vi "GUIAS CURVAS EM FUNÇÃO DO RAIO-6.vi"() -> ()   [LabVIEW 2014]
uses:
  <vilib>/Platform/TimedLoop/XDataNode/timing_clust.ctl
  <vilib>/Platform/TimedLoop/XDataNode/nitl_modes.ctl
  <vilib>/Platform/TimedLoop/XDataNode/wakeup.ctl
  <vilib>/Instr/_visa.llb/VISA Configure Serial Port (Instr).vi
  <vilib>/Platform/TimedLoop/XDataNode/XDataNode.xnode
  <userlib>/Newport ESP301/Newport ESP301.lvlib
  <vilib>/Platform/TimedLoop/XDataNode/XDNodeRunTimeDep.lvlib
panel:
  in  "Aceleracao":dbl=2.0
  in  "Velocity":dbl=3.0
  out "Yin":dbl format="%.6g"
  out "Xin":dbl format="%.6g"
  out "Raio":dbl
  out "PROGRESSÃO":i32
  in  "Raios":dbl[](array[numeric])=[40.0, 60.0, 80.0, 100.0, 120.0, 140.0, 180.0]
  in  "N_Guias":dbl=7.0
  in  "Iniciar":bool
  in  "L":dbl=10.0 format="%.1f"
  in  "In.Curva":dbl=2.0
  out "d (um)":dbl
  in  "Distância (um)":dbl=50.0
  in  "Stop Button":bool
  out "X (mm)":dbl format="%.2g"
  out "Y (um)":dbl format="%.1f"
  out "XY Graph":cluster{dbl[], dbl[]}(graph)={[0.0, 0.0, 0.0, 0.0, 0.0, 0.0, 0.0, 0.0, 0.0, 0.0, 0.0, 0.0, 0.0, 0.0, 0.0, 0.0, 0.0, 0.0, 0.0, 0.0, 0.0, 0.0, 0.0, 0.0, 0.0, 0.0, 0.0, 0.0, 0.0, 0.0, 0.0, 0.0, 0.0, 0.0, 0.0, 0.0, 0.0, 0.0, 0.0, 0.0, 0.0, 0.0, 0.0, 0.0, 0.0, 0.0, 0.0, 0.0, 0.0, 0.0, 0.0, 0.0, 0.0, 0.0, 0.0, 0.0, 0.0, 0.0, 0.0, 0.0, 0.0, 0.0, 0.0, 0.0, 0.0, 0.0, 0.0, 0.0, 0.0, 0.0, 0.0, 0.0, 0.0, 0.0, 0.0, 0.0], [4600.0, 4600.0, 4600.0, 4600.0, 4600.0, 4600.0, 4600.0, 4600.0, 4600.0, 4600.0, 4600.0, 4600.0, 4600.0, 4600.0, 4600.0, 4600.0, 4600.0, 4600.0, 4600.0, 4600.0, 4600.0, 4600.0, 4600.0, 4600.0, 4600.0, 4600.0, 4600.0, 4690.0, 4802.5, 4800.5, 4799.5, 4799.5, 4799.5, 4800.0, 4800.0, 4800.0, 4800.0, 4800.0, 4800.0, 4800.0, 4800.0, 4800.0, 4800.0, 4800.0, 4995.5, 5001.5, 5000.5, 5000.0, 5000.0, 4999.5, 4999.5, 5000.0, 5000.0, 5000.0, 5000.0, 5000.0, 5000.0, 5000.0, 5000.0, 5000.0, 5000.0, 5000.0, 5000.0, 5000.0, 5000.0, 5000.0, 5000.0, 5000.0, 5000.0, 5000.0, 5000.0, 5000.0, 5000.0, 5000.0, 5000.0, 5000.0]}
  in  "Refresh Button":bool
  # "Inicio curva"
  # "Tam.amostra (mm)"
  # "Núm.guias"
  # "Raio (mm)"
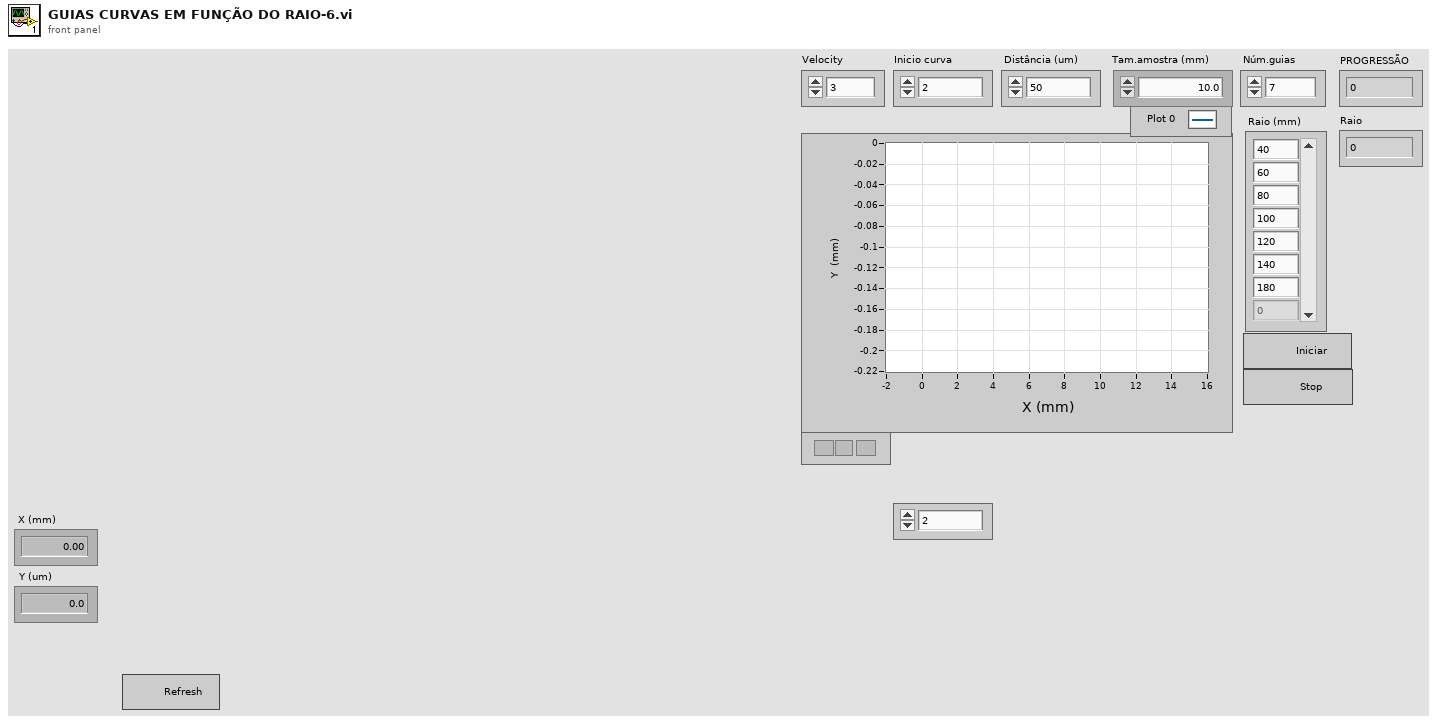
[diagram p1: front panel]
types:
  T1 = typedef "XDNodeRunTimeDep.lvlib/timing_clust.ctl" = cluster{"Expected End [f-1]":u64, "Actual End [f-1]":u64, "Finished Late? [f-1]":bool, "Expected End [i-1]":u64, "Actual End [i-1]":u64, "Finished Late? [i-1]":bool, "Expected Start [i]":u64, "Actual Start [i]":u64, "Expected Start [f]":u64, "Actual Start [f]":u64, "Source Name":string, "Structure Name":string, "Period":i64, "Deadline":i64, "Offset":i64, "Start":i64, "Priority":i32, "Timeout":i32, "Mode":T2, "Wakeup Reason":T3, "Error":errorcluster, "Source Type":string, "Secondary Source Type":string, "Global End Time":u64, "Global Start Time":u64, "Frame Duration":u64, "Iteration Duration":u64, "Assigned CPU":i32, "I/O Scan Engine Mode":u32}
  T2 = typedef "XDNodeRunTimeDep.lvlib/nitl_modes.ctl" = enum32{"No Change", "Process missed periods, maintain original phase", "Discard missed periods, maintain original phase", "Process missed periods, ignore original phase", "Discard missed periods, ignore original phase"}
  T3 = typedef "XDNodeRunTimeDep.lvlib/wakeup.ctl" = enum32{"Normal", "Aborted", "Asynchronous wakeup", "Timing source error", "Timed loop error", "Timeout"}
  T4 = cluster{"Axis1 moving":bool, "Axis2 moving":bool, "Axis3 moving":bool, "Axis4 moving":bool, "Motor Power of at least one axis":bool, "Reserved":bool, "Reserved":bool, "Reserved":bool, "Axis5 moving 2":bool, "Axis6 moving 2":bool, "Reserved":bool, "Reserved":bool, "Motor Power of at least one axis":bool, "Reserved":bool, "Reserved":bool, "Reserved":bool}
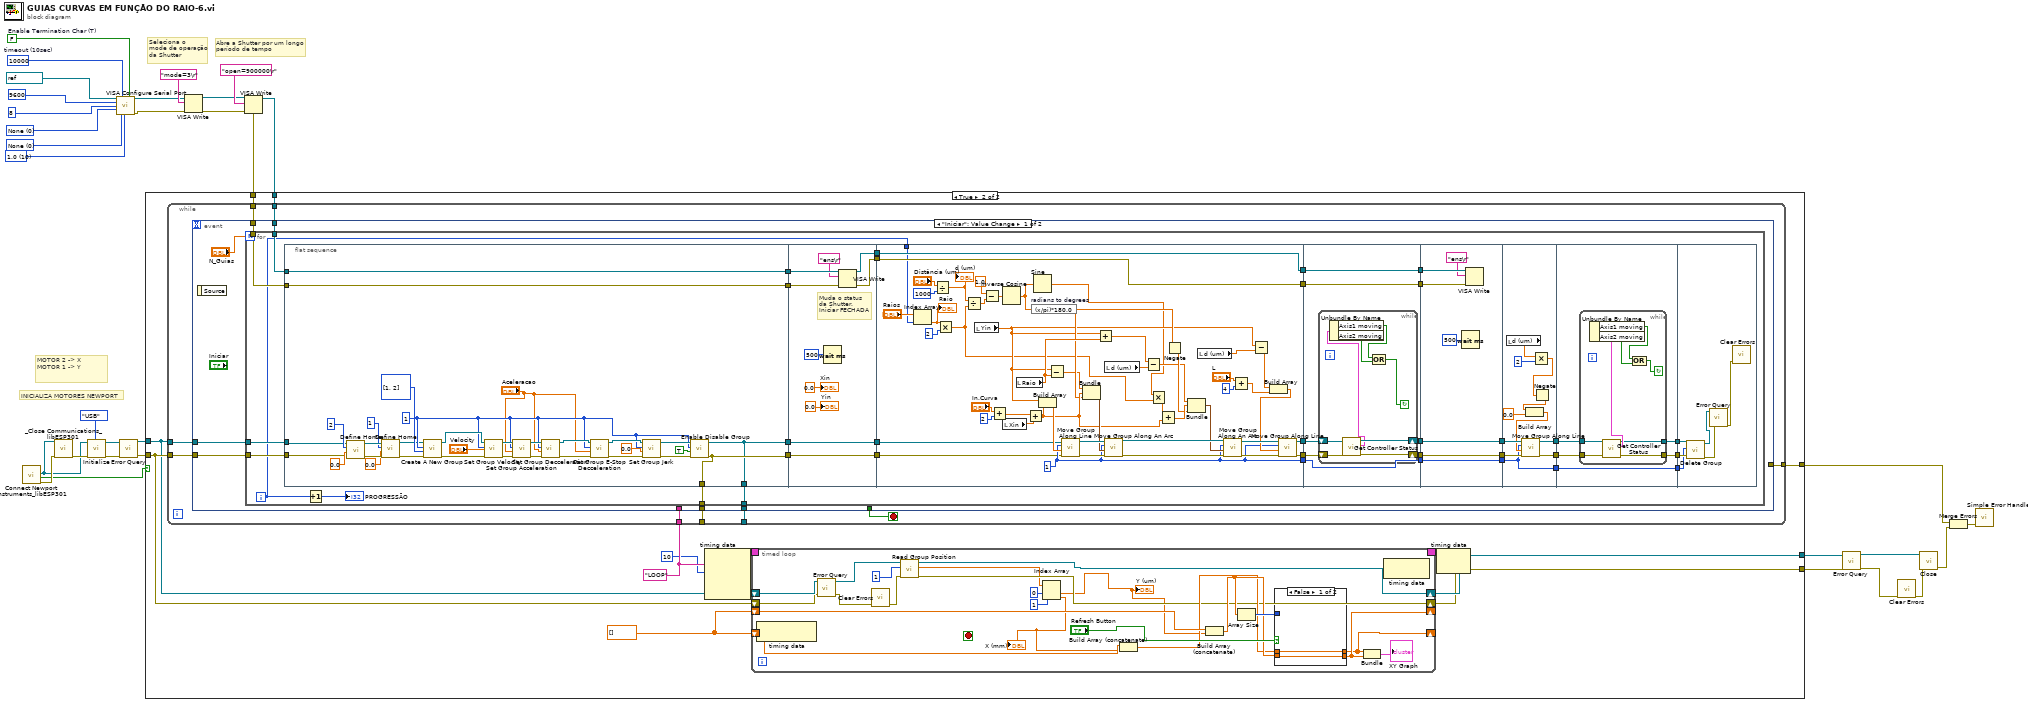
[diagram p0: block diagram]
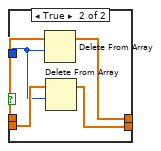
[diagram p3: hidden frame]
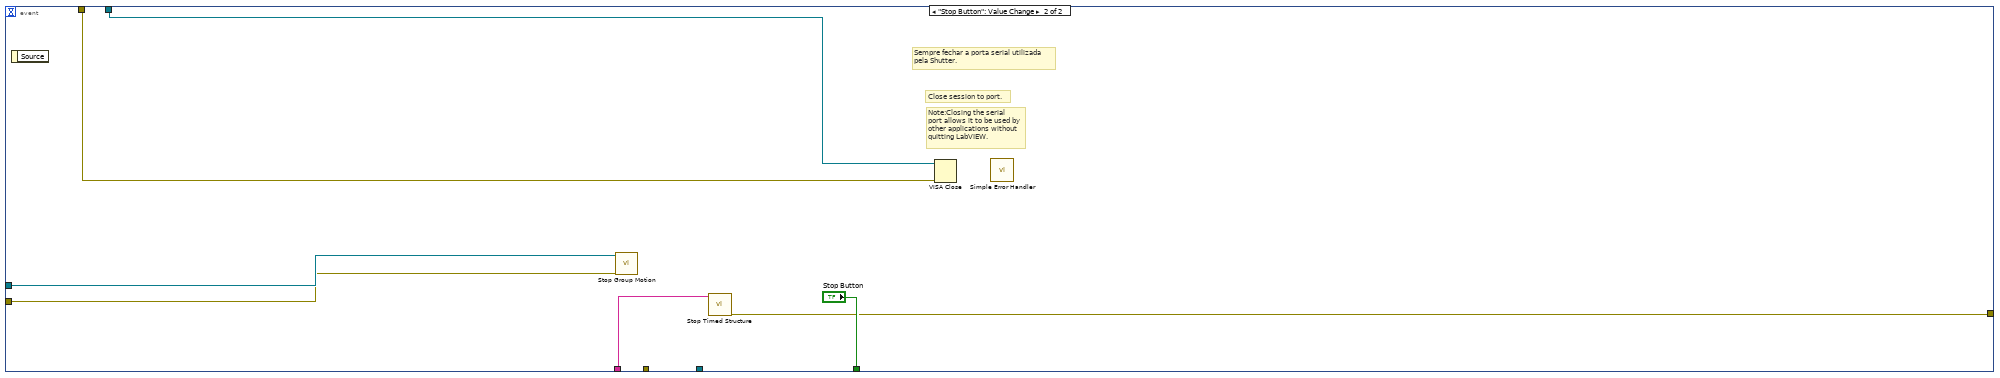
[diagram p4: hidden frame]
diagram:
  w9 = u16 0 items=["None", "Odd", "Even", "Mark", "Space"] ("parity")
  w12 = u16 10 items=["1.0"=10, "1.5"=15, "2.0"=20] ("stop bits")
  w13 = u16 0 items=["None"=0, "XON/XOFF"=1, "RTS/CTS"=2, "DTR/DSR"=4] ("flow control")
  w11 = FALSE  # Enable Termination Char (T)
  w10 = u32 10000  # timeout (10sec)
  # "Abre a Shutter por um longo\nperíodo de tempo"
  # "Seleciona o \nmode de operação\nda Shutter"
  # "MOTOR 2 -> X\nMOTOR 1 -> Y"
  # "INICIALIZA MOTORES NEWPORT"
  n1 = call <userlib>:"Connect Newport Instruments_libESP301.vi"() -> ("error (duplicate)"=w31:errorcluster, "Connected"=w20:bool, "VISA resource name (duplicate)"=w30:refnum<visa-resource-name>)  [unwired: 7 in, 2 out]
  n2 = call <userlib>:"_Close Communications_libESP301.vi"("Instrument Channel"=w30, "error in (no error)"=w31) -> ("error out"=w33:errorcluster)  [unwired: 13 in]
  n3 = call <userlib>:"Initialize.vi"("VISA resource name"=w30, "error in (no error)"=w33, "Serial Link (RS232)"=enum16{"RS232", "USB"}."USB") -> ("VISA resource name out"=w29:refnum<visa-resource-name>, "error out"=w28:errorcluster)  [unwired: 6 in]
  n4 = call-poly "VISA Configure Serial Port"("VISA resource name"=refnum<visa-resource-name> "COM6", "timeout (10sec)"=w10, "Enable Termination\nChar (T)"=w11, "baud rate (9600)"=u32 9600 ("baud rate"), "data bits (8)"=u16 8 ("data bits"), "parity (0:none)"=w9, "stop bits (10: 1 bit)"=w12, "flow control (0:none)"=w13) -> ("VISA resource name out"=w5:refnum<visa-resource-name>, "error out"=w4:errorcluster)  [unwired: 6 in]
  n5 = call <userlib>:"Error Query.vi"("error in (no error)"=w28, "VISA resource name"=w29) -> ("error out"=w17:errorcluster, "VISA resource name out"=w18:refnum<visa-resource-name>)  [unwired: 2 in, 2 out]
  n6 = VISA Write(VISA resource name=w5, write buffer="mode=3\r", error in (no error)=w4) -> (VISA resource name out=w2:refnum<visa-resource-name>, error out=w1:errorcluster)  [unwired: 1 out]
  n7 = VISA Write(VISA resource name=w2, write buffer="open=900000\r", error in (no error)=w1) -> (VISA resource name out=w21:refnum<visa-resource-name>, error out=w19:errorcluster)  [unwired: 1 out]
  n8 = case shown="True" w20 {
    tunnel: [w35 w47] -> w16
    tunnel: [w34 w46] -> w15
    tunnel: w18 -> [w35 w36]
    tunnel: w17 -> [w34 w37]
    tunnel: [_ w44] -> w24
    tunnel: w21 -> [_ w43]
    tunnel: w19 -> [_ w42]
    frame False {
    }
    frame True {
      w38 = dbl[] []
      w45 = "LOOP" ("Structure Name")
      n9 = while {
        tunnel: w37 -> [w92]
        tunnel: w36 -> [w91]
        tunnel: w45 -> [w89]
        tunnel: [w88] -> w44
        tunnel: w43 -> [w87]
        tunnel: w42 -> [w86]
        tunnel: [w85] -> _
        tunnel: [w84] -> _
        stop <- w90 stop-if-true
        n10 = event shown="[0] \"Iniciar\": Value Change" {
          selector: _ -> [_ _]
          dyn-events: _ -> [_ _]
          timeout: _ -> [_ _]
          tunnel: w92 -> [w99 w280]
          tunnel: w91 -> [w98 w281]
          tunnel: [_ "Stop Button"] -> w90
          tunnel: w89 -> [_ w284]
          tunnel: [_ w283] -> w88
          tunnel: w87 -> [w96 w282]
          tunnel: w86 -> [w95 w279]
          tunnel: [w94 _] -> w85
          tunnel: [w93 _] -> w84
          event "Iniciar": Value Change {
            n11 = event-data() -> ()  [unwired: 1 in, 1 out]
            n12 = for {
              N: "N_Guias" -> [_]
              tunnel: w99 -> [w132]
              tunnel: w98 -> [w131]
              tunnel: w96 -> [w129]
              tunnel: w95 -> [w111]
              tunnel: [w101] -> w94
              tunnel: [w100] -> w93
              i -> [w110]
              n13 = flat-sequence {
                tunnel: w111 -> [w165]
                tunnel: w129 -> [w166]
                tunnel: w131 -> [w139]
                tunnel: w132 -> [w138]
                tunnel: [w137] -> w109
                tunnel: [w136] -> w108
                tunnel: [w166] -> w107
                tunnel: [w165] -> w106
                tunnel: [w137] -> w101
                tunnel: [w136] -> w100
                tunnel: [w170] -> w134
                tunnel: [w171] -> w133
                tunnel: [w174] -> w119
                tunnel: [w173] -> w116
                tunnel: w109 -> [w170]
                tunnel: w108 -> [w171]
                tunnel: w107 -> [w175]
                tunnel: w106 -> [w172]
                tunnel: w134 -> [w179]
                tunnel: w133 -> [w180]
                tunnel: w110 -> [w188]
                tunnel: [w193] -> w126
                tunnel: [w192] -> w125
                tunnel: [w191] -> w122
                tunnel: w119 -> [w189]
                tunnel: [w190] -> w117
                tunnel: w116 -> [w190]
                tunnel: [w189] -> w115
                tunnel: [w233] -> w127
                tunnel: w126 -> [w233]
                tunnel: w125 -> [w229]
                tunnel: [w227] -> w124
                tunnel: w122 -> [w230]
                tunnel: [w228] -> w121
                tunnel: [w232] -> w118
                tunnel: w117 -> [w232]
                tunnel: w115 -> [w231]
                tunnel: [w231] -> w114
                tunnel: [w248] -> w128
                tunnel: w127 -> [w248]
                tunnel: w124 -> [w247]
                tunnel: [w247] -> w123
                tunnel: w121 -> [w246]
                tunnel: [w246] -> w120
                tunnel: w118 -> [w245]
                tunnel: w114 -> [w244]
                tunnel: w128 -> [w249]
                tunnel: w123 -> [w259]
                tunnel: w120 -> [w258]
                tunnel: [w252] -> w113
                tunnel: [w251] -> w112
                tunnel: [w249] -> w102
                tunnel: w113 -> [w264]
                tunnel: w112 -> [w263]
                tunnel: [w262] -> w105
                tunnel: [w261] -> w104
                tunnel: [w260] -> w103
                tunnel: w102 -> [w260]
                tunnel: w105 -> [w278]
                tunnel: w104 -> [w277]
                tunnel: w103 -> [w276]
                frame #0 {
                  w148 = 1 ("Group #")
                  n14 = call <userlib>:"Define Home.vi"("error in (no error)"=w138, "Home Position (0 units)"=0.0, "Axis (1)"=2 ("y"), "VISA resource name"=w139) -> ("error out"=w146:errorcluster, "VISA resource name out"=w147:refnum<visa-resource-name>)  [unwired: 2 in]
                  n15 = call <userlib>:"Define Home.vi"("error in (no error)"=w146, "Home Position (0 units)"=0.0, "Axis (1)"=1, "VISA resource name"=w147) -> ("error out"=w140:errorcluster, "VISA resource name out"=w141:refnum<visa-resource-name>)  [unwired: 2 in]
                  n16 = call <userlib>:"Create A New Group.vi"("error in (no error)"=w140, "Axis Number"=i32[] [1, 2], "Group Number (1)"=w148, "VISA resource name"=w141) -> ("error out"=w162:errorcluster, "VISA resource name out"=w163:refnum<visa-resource-name>)  [unwired: 2 in]
                  n17 = call <userlib>:"Set Group Velocity.vi"("error in (no error)"=w162, "Velocity (units/s)"="Velocity", "Group Number (1)"=w148, "VISA resource name"=w163) -> ("error out"=w157:errorcluster, "VISA resource name out"=w160:refnum<visa-resource-name>)  [unwired: 2 in]
                  n18 = call <userlib>:"Set Group Acceleration.vi"("error in (no error)"=w157, "Acceleration (0 units/s²)"="Aceleracao", "Group Number (1)"=w148, "VISA resource name"=w160) -> ("error out"=w158:errorcluster, "VISA resource name out"=w159:refnum<visa-resource-name>)  [unwired: 2 in]
                  n19 = call <userlib>:"Set Group Decceleration.vi"("error in (no error)"=w158, "Decceleration (0 units/s²)"="Aceleracao", "Group Number (1)"=w148, "VISA resource name"=w159) -> ("error out"=w153:errorcluster, "VISA resource name out"=w156:refnum<visa-resource-name>)  [unwired: 2 in]
                  n20 = call <userlib>:"Set Group E-Stop Decceleration.vi"("error in (no error)"=w153, "E-Stop Decceleration (0 units/s²)"="Aceleracao", "Group Number (1)"=w148, "VISA resource name"=w156) -> ("error out"=w152:errorcluster, "VISA resource name out"=w155:refnum<visa-resource-name>)  [unwired: 2 in]
                  n21 = call <userlib>:"Set Group Jerk.vi"("error in (no error)"=w152, "Vector Jerk (0 units/s^3)"=0.0, "Group Number (1)"=w148, "VISA resource name"=w155) -> ("error out"=w151:errorcluster, "VISA resource name out"=w154:refnum<visa-resource-name>)  [unwired: 2 in]
                  n22 = call <userlib>:"Enable Disable Group.vi"("error in (no error)"=w151, "Action (OFF)"=TRUE, "Group Number (1)"=w148, "VISA resource name"=w154) -> ("error out"=w137:errorcluster, "VISA resource name out"=w136:refnum<visa-resource-name>)  [unwired: 2 in]
                }
                frame #1 {
                  # "Muda o status\nda Shutter.\nIniciar FECHADA"
                  n23 = Wait (ms)(milliseconds to wait=u32 500) -> ()  [unwired: 1 out]
                  n24 = VISA Write(VISA resource name=w175, write buffer="ens\r", error in (no error)=w172) -> (VISA resource name out=w174:refnum<visa-resource-name>, error out=w173:errorcluster)  [unwired: 1 out]
                  "Xin" <- 0.0 ("Xin")
                  "Yin" <- 0.0 ("Yin")
                }
                frame #2 {
                  w193 = 1 ("y")
                  n25 = Index Array(array="Raios", index=w188) -> (element=w194:dbl)
                  "Raio" <- w194
                  n26 = Divide(x="Distância (um)", y=1000) -> (x/y=w217:dbl)
                  "d (um)" <- w217
                  n27 = Multiply(x=w194, y=2) -> (x*y=w178:dbl)
                  n28 = Divide(x=w217, y=w178) -> (x/y=w220:dbl)
                  n29 = local read "Yin"() -> (w186:dbl)
                  n30 = Subtract(x=1.0, y=w220) -> (x-y=w218:dbl)
                  n31 = Add(x="In.Curva", y=2) -> (x+y=w206:dbl)
                  n32 = Inverse Cosine(1:w218) -> (0:w207:dbl)
                  n33 = local read "Xin"() -> (w208:dbl)
                  n34 = local read "Raio"() -> (w202:dbl)
                  n35 = Add(x=w206, y=w208) -> (x+y=w204:dbl)
                  n36 = expression code="(x/pi)*180.0" "radians to degrees"(w207) -> (w198:dbl)
                  n37 = Sine(x=w207) -> (sin(x)=w177:dbl)
                  n38 = Build Array(w186, w204) -> (w214:dbl[])
                  n39 = Subtract(x=w186, y=w202) -> (x-y=w185:dbl)
                  n40 = call <userlib>:"Move Group Along Line.vi"("error in (no error)"=w179, "Position (0 units)"=w214, "Group Number (1)"=w193, "VISA resource name"=w180) -> ("error out"=w212:errorcluster, "VISA resource name out"=w213:refnum<visa-resource-name>)  [unwired: 2 in]
                  n41 = Bundle(w185, w204, w198) -> (w211:cluster{dbl, dbl, dbl})  [unwired: 1 in]
                  n42 = Add(x=w186, y=w202) -> (x+y=w182:dbl)
                  n43 = local read "d (um)"() -> (w183:dbl)
                  n44 = call <userlib>:"Move Group Along An Arc.vi"("error in (no error)"=w212, "Arc  Parameters"=w211, "Group Number (1)"=w193, "VISA resource name"=w213) -> ("error out"=w225:errorcluster, "VISA resource name out"=w226:refnum<visa-resource-name>)  [unwired: 2 in]
                  n45 = Subtract(x=w182, y=w183) -> (x-y=w181:dbl)
                  n46 = Multiply(x=w177, y=w178) -> (x*y=w205:dbl)
                  n47 = Add(x=w205, y=w204) -> (x+y=w203:dbl)
                  n48 = Negate(x=w198) -> (-x=w197:dbl)
                  n49 = Bundle(w181, w203, w197) -> (w224:cluster{dbl, dbl, dbl})  [unwired: 1 in]
                  n50 = local read "d (um)"() -> (w184:dbl)
                  n51 = call <userlib>:"Move Group Along An Arc.vi"("error in (no error)"=w225, "Arc  Parameters"=w224, "Group Number (1)"=w193, "VISA resource name"=w226) -> ("error out"=w196:errorcluster, "VISA resource name out"=w201:refnum<visa-resource-name>)  [unwired: 2 in]
                  n52 = Add(x="L", y=4) -> (x+y=w200:dbl)
                  n53 = Subtract(x=w186, y=w184) -> (x-y=w187:dbl)
                  n54 = Build Array(w187, w200) -> (w199:dbl[])
                  n55 = call <userlib>:"Move Group Along Line.vi"("error in (no error)"=w196, "Position (0 units)"=w199, "Group Number (1)"=w193, "VISA resource name"=w201) -> ("error out"=w192:errorcluster, "VISA resource name out"=w191:refnum<visa-resource-name>)  [unwired: 2 in]
                }
                frame #3 {
                  n56 = while {
                    shift-right: [w237] -> w228
                    shift-left: w230 -> [w239]
                    shift-right: [w236] -> w227
                    shift-left: w229 -> [w238]
                    stop <- w234 continue-if-true
                    n57 = call <userlib>:"Get Controller Status.vi"("error in (no error)"=w238, "VISA resource name"=w239) -> ("error out"=w236:errorcluster, "Controller Status"=w235:T4, "VISA resource name out"=w237:refnum<visa-resource-name>)  [unwired: 2 in, 1 out]
                    n58 = Unbundle By Name(w235) -> ("Axis1 moving"=w241:bool, "Axis2 moving"=w240:bool)
                    n59 = Compound Arithmetic op=OR(w241, w240) -> (w234:bool)
                  }
                }
                frame #4 {
                  n60 = Wait (ms)(milliseconds to wait=u32 500) -> ()  [unwired: 1 out]
                  n61 = VISA Write(VISA resource name=w244, write buffer="ens\r", error in (no error)=w245) -> ()  [unwired: 3 out]
                }
                frame #5 {
                  n62 = local read "d (um)"() -> (w255:dbl)
                  n63 = Multiply(x=w255, y=2) -> (x*y=w250:dbl)
                  n64 = Negate(x=w250) -> (-x=w253:dbl)
                  n65 = Build Array(w253, 0.0 ("element")) -> (w257:dbl[])
                  n66 = call <userlib>:"Move Group Along Line.vi"("error in (no error)"=w259, "Position (0 units)"=w257, "Group Number (1)"=w249, "VISA resource name"=w258) -> ("error out"=w251:errorcluster, "VISA resource name out"=w252:refnum<visa-resource-name>)  [unwired: 2 in]
                }
                frame #6 {
                  n67 = while {
                    tunnel: w264 -> [w268]
                    tunnel: w263 -> [w267]
                    tunnel: [w266] -> w262
                    tunnel: [w265] -> w261
                    stop <- w269 continue-if-true
                    n68 = call <userlib>:"Get Controller Status.vi"("error in (no error)"=w267, "VISA resource name"=w268) -> ("error out"=w265:errorcluster, "Controller Status"=w272:T4, "VISA resource name out"=w266:refnum<visa-resource-name>)  [unwired: 2 in, 1 out]
                    n69 = Unbundle By Name(w272) -> ("Axis1 moving"=w271:bool, "Axis2 moving"=w270:bool)
                    n70 = Compound Arithmetic op=OR(w271, w270) -> (w269:bool)
                  }
                }
                frame #7 {
                  n71 = call <userlib>:"Delete Group.vi"("error in (no error)"=w277, "Group Number (1)"=w276, "VISA resource name"=w278) -> ("error out"=w273:errorcluster, "VISA resource name out"=w274:refnum<visa-resource-name>)  [unwired: 3 in]
                  n72 = call <userlib>:"Error Query.vi"("error in (no error)"=w273, "VISA resource name"=w274) -> ("error out"=w275:errorcluster)  [unwired: 2 in, 3 out]
                  n73 = call <vilib>:"Clear Errors.vi"("error in (no error)"=w275) -> ()  [unwired: 5 in, 2 out]
                }
              }
              n74 = Increment(x=w110) -> (x+1=→"PROGRESSÃO":i32)
            }
          }
          event "Stop Button": Value Change {
            # "Sempre fechar a porta serial utilizada\npela Shutter."
            # "Note:Closing the serial port allows it to be used by other applications without\nquitting LabVIEW."
            # "Close session to port."
            n75 = event-data() -> ()  [unwired: 1 in, 1 out]
            n76 = call <userlib>:"Stop Group Motion.vi"("error in (no error)"=w280, "VISA resource name"=w281) -> ()  [unwired: 4 in, 2 out]
            n77 = call <vilib>:"Stop Timed Structure.vi"("name"=w284) -> ("error out"=w283:errorcluster)  [unwired: 10 in]
            n78 = VISA Close(VISA resource name=w282, error in (no error)=w279) -> ()  [unwired: 1 out]
            n79 = call <vilib>:"Simple Error Handler.vi"() -> ()  [unwired: 5 in, 5 out]
          }
        }
      }
      n80 = node-c288(w45, i64 10 ("Period")) -> (w41:T1)  [unwired: 2 in]
      n81 = timed-loop {
        timing: w41 -> [_]
        timing-out: [_] -> w40
        shift-right: [w59] -> w47
        shift-left: w36 -> [w52]
        shift-right: [w58] -> w46
        shift-left: w37 -> [w51]
        shift-right: [w62] -> _
        shift-left: w38 -> [w66]
        shift-right: [w61] -> _
        shift-left: w38 -> [w64]
        stop <- _ stop-if-true
        n82 = node-c288() -> ()  [unwired: 1 in, 1 out]
        n83 = call <userlib>:"Error Query.vi"("error in (no error)"=w51, "VISA resource name"=w52) -> ("error out"=w49:errorcluster, "VISA resource name out"=w50:refnum<visa-resource-name>)  [unwired: 2 in, 2 out]
        n84 = call <vilib>:"Clear Errors.vi"("error in (no error)"=w49) -> ("error out"=w48:errorcluster)  [unwired: 5 in, 1 out]
        n85 = call <userlib>:"Read Group Position.vi"("error in (no error)"=w48, "Group Number (1)"=1, "VISA resource name"=w50) -> ("error out"=w58:errorcluster, "Position (units)"=w55:dbl[], "VISA resource name out"=w59:refnum<visa-resource-name>)  [unwired: 2 in]
        n86 = Index Array(array=w55, index #1=0 ("index"), index #2=1 ("index")) -> (element #1=w54:dbl, element #2=w53:dbl)
        "X (mm)" <- w53
        "Y (um)" <- w54
        n87 = Build Array (concatenate)(w64, w53) -> (w63:dbl[])
        n88 = Build Array (concatenate)(w66, w54) -> (w65:dbl[])
        n89 = Array Size(array=w65) -> (size(s)=w67:i32)
        n90 = case shown="False" "Refresh Button" {
          tunnel: [w71 w73] -> w61
          tunnel: w63 -> [w71 w76]
          tunnel: [w70 w72] -> w62
          tunnel: w65 -> [w70 w75]
          tunnel: w67 -> [_ w74]
          frame False {
          }
          frame True {
            n91 = Delete From Array(array=w76, length=w74) -> (array with subset deleted=w73:dbl[])  [unwired: 1 in, 1 out]
            n92 = Delete From Array(array=w75, length=w74) -> (array with subset deleted=w72:dbl[])  [unwired: 1 in, 1 out]
          }
        }
        n93 = Bundle(w61, w62) -> (→"XY Graph":cluster{dbl[], dbl[]})  [unwired: 1 in]
        n94 = node-c288() -> ()  [unwired: 1 in, 1 out]
      }
      n95 = node-c288(w40) -> ()  [unwired: 1 out]
    }
  }
  n96 = call <userlib>:"Error Query.vi"("error in (no error)"=w15, "VISA resource name"=w16) -> ("error out"=w25:errorcluster, "VISA resource name out"=w26:refnum<visa-resource-name>)  [unwired: 2 in, 2 out]
  n97 = call <vilib>:"Clear Errors.vi"("error in (no error)"=w25) -> ("error out"=w27:errorcluster)  [unwired: 5 in, 1 out]
  n98 = call <userlib>:"Close.vi"("error in (no error)"=w27, "VISA resource name"=w26) -> ("error out"=w23:errorcluster)  [unwired: 9 in]
  n99 = Merge Errors(w24, w23) -> (w22:errorcluster)
  n100 = call <vilib>:"Simple Error Handler.vi"("error in (no error)"=w22) -> ()  [unwired: 4 in, 5 out]
